vi "CheckOutputData.vi"(8 "error in (no error)":errorcluster, 11 "OutputData":waveform(dbl)) -> (0 "error out":errorcluster, 3 "Empty":bool)   [LabVIEW 2022 SP3]
uses:
  <vilib>/Waveform/WDTOps.llb/WDT Number of Waveform Samples DBL.vi
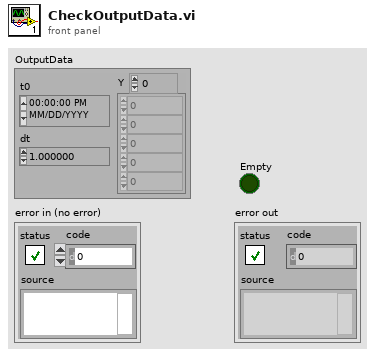
[diagram p1: front panel]
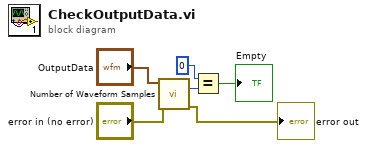
[diagram p0: block diagram]
diagram:
  n1 = call-poly <vilib>:"Number of Waveform Samples.vi"("error in (no error)"="error in (no error)", "waveform in"="OutputData") -> ("error out"=→"error out":errorcluster, "number of samples"=w6:i32)  [unwired: 7 in, 1 out]
  n2 = Equal?(x=0, y=w6) -> (x = y?=→"Empty":bool)
